vi "DAC Run.vi"(8 "error in":errorcluster, 11 "DAC HTS dU in":refnum<class "DAC HTS dU.lvclass">) -> (0 "error out":errorcluster, 3 "DAC HTS dU out":refnum<class "DAC HTS dU.lvclass">)   [LabVIEW 2019, in "DAC.lvlib" / "DAC HTS dU.lvclass"]
uses:
  DAC HTS dU.lvclass
  C:/Users/krio/Documents/LV_Projects/test-stand/App/DAC/DAC.lvclass
  DAC.lvclass/DAC.ctl
  Results/HTS Results/HTS Results.lvclass
  Results/Results Method.ctl
  DAC HTS dU.lvclass/DAC HTS dU.ctl
  Results/HTS Results/HTS Results.lvclass/HTS Results.ctl
  <vilib>/regexp/Match Regular Expression.xnode
  DAC.lvclass
  Results/Results.lvlib
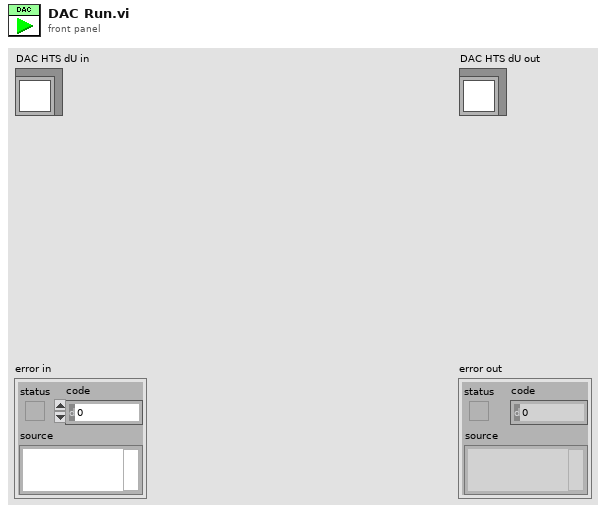
[diagram p1: front panel]
types:
  T1 = typedef "Results.lvlib/Results Method.ctl" = enum16{"Get", "Set"}
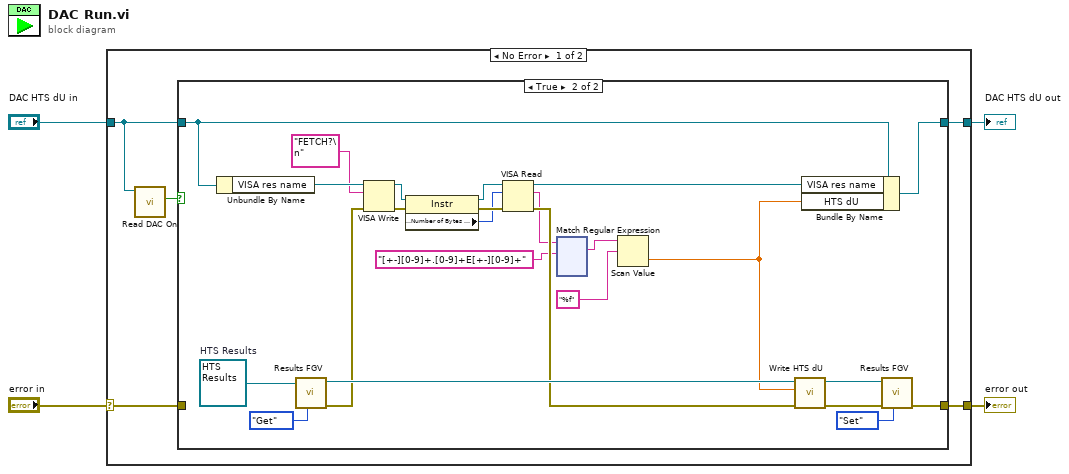
[diagram p0: block diagram]
diagram:
  n1 = case shown="No Error" "error in" {
    selector: "error in" -> [w7 w151]
    tunnel: [w6 w151] -> w2
    tunnel: [w8 w150] -> w1
    tunnel: "DAC HTS dU in" -> [w5 w150]
    frame No Error {
      n2 = call "Read DAC On.vi"("DAC in"=w5) -> ("DAC On"=w9:bool)  [unwired: 8 in, 2 out]
      n3 = case shown="True" w9 {
        tunnel: w5 -> [w11 w35]
        tunnel: [w11 w31] -> w8
        tunnel: w7 -> [w10 _]
        tunnel: [w10 w30] -> w6
        frame False {
        }
        frame True {
          w34 = refnum<class "HTS Results.lvclass"> refnum  # HTS Results
          n4 = Unbundle By Name(w35) -> ("VISA res name"=w24:refnum<visa-resource-name>)
          n5 = call-dynamic "Results FGV.vi"("Method"=Results_Method."Get", "HTS Results in"=w34) -> ("error out"=w22:errorcluster, "HTS Results out"=w29:refnum<class "HTS Results.lvclass">)  [unwired: 8 in]
          n6 = VISA Write(VISA resource name=w24, write buffer="FETCH?\n", error in (no error)=w22) -> (VISA resource name out=w15:refnum<visa-resource-name>, error out=w17:errorcluster)  [unwired: 1 out]
          n7 = property class="Instr"(reference=w15, error in=w17) -> (reference out=w26:refnum<visa-resource-name>, error out=w25:errorcluster, "Serial Settings:Number of Bytes at Serial Port"=w16:u32)
          n8 = VISA Read(VISA resource name=w26, byte count=w16, error in (no error)=w25) -> (VISA resource name out=w19:refnum<visa-resource-name>, read buffer=w14:string, error out=w18:errorcluster)  [unwired: 1 out]
          n9 = xnode "Match Regular Expression"("input string"=w14, "regular expression"="[+-][0-9]+.[0-9]+E[+-][0-9]+") -> ("whole match"=w13:string)  [unwired: 4 in, 4 out]
          n10 = Scan Value(string=w13, format string="%f") -> (value=w20:dbl)  [unwired: 1 in, 1 out]
          n11 = call "Write HTS dU.vi"("error in (no error)"=w18, "HTS dU"=w20, "HTS Results in"=w29) -> ("error out"=w27:errorcluster, "HTS Results out"=w28:refnum<class "HTS Results.lvclass">)  [unwired: 7 in]
          n12 = Bundle By Name(cluster=w35, "VISA res name"=w19, "HTS dU"=w20) -> (w31:refnum<class "DAC HTS dU.lvclass">)
          n13 = call-dynamic "Results FGV.vi"("Method"=Results_Method."Set", "error in"=w27, "HTS Results in"=w28) -> ("error out"=w30:errorcluster)  [unwired: 7 in, 1 out]
        }
      }
    }
    frame Error {
    }
  }
  "error out" <- w2
  "DAC HTS dU out" <- w1
